vi "WM JONSWAP.vi"(3 "Sigma B":dbl=0.09 format="%.2f", 4 "End Freq (Model Scale)":dbl=100.0 min=0.0 format="%.2f", 5 "Start Freq (Model Scale)":dbl min=0.0 format="%.2f", 6 "Gamma":dbl=3.3 min=-1.0 max=9.0 format="%.2f", 7 "Sigma A":dbl=0.07 format="%.2f", 8 "Number of Frequencies":i32=100 min=2, 9 "Scale Ratio":dbl=1.0 min=0.0 step=0.01 format="%.2f", 10 "Peak Wave Period":dbl=1.0 min=0.0 step=0.01 format="%.2f", 11 "Significant Wave Height":dbl=1.0 min=0.0 step=0.01 format="%.2f") -> (0 "Frequency":dbl[](array[numeric]) caption="Hz" format="%.2f", 1 "Spectral Energy":dbl[](array[numeric]) format="%.2f", 2 "JONSWAP parameters":T1 {"Scale Ratio" format="%.2f"; "Sigma B" format="%.2f"; "Sigma A" format="%.2f"; "Gamma" format="%.2f"; "Sig Wave Period" format="%.2f"; "Sig Wave Height" format="%.2f"})   [LabVIEW 2012]
panel:
  in  "Boolean":bool
  # "JONSWAP Wave Spectra"
  # "m  (Full Scale)"
  # "s  (Full Scale)"
  # ":1"
  # "Full Scale : Model Scale"
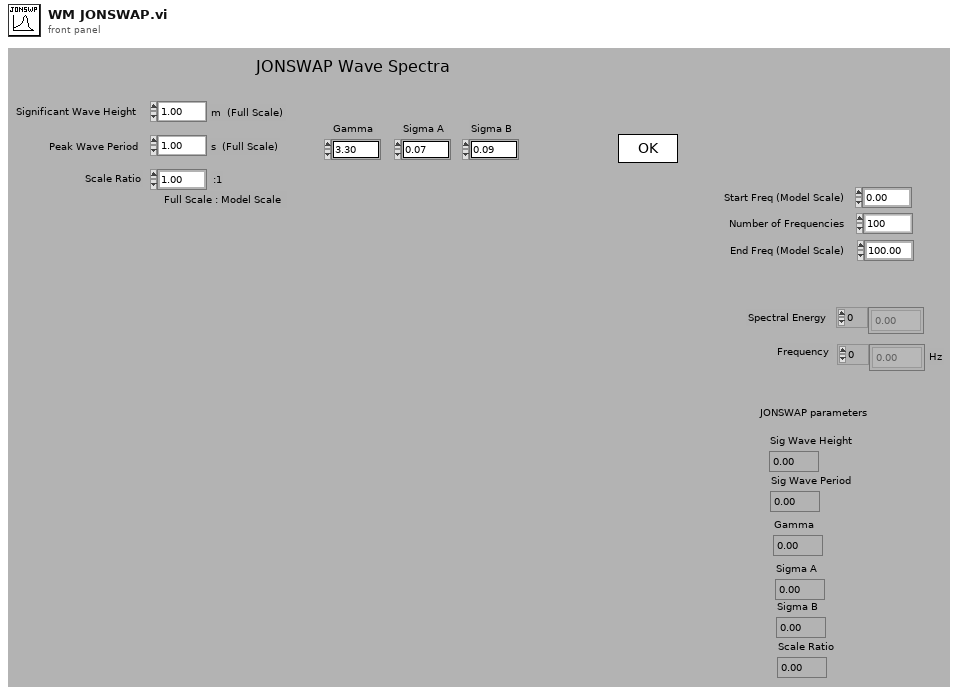
[diagram p1: front panel]
types:
  T1 = cluster{"Sig Wave Height":dbl, "Sig Wave Period":dbl, "Gamma":dbl, "Sigma A":dbl, "Sigma B":dbl, "Scale Ratio":dbl}
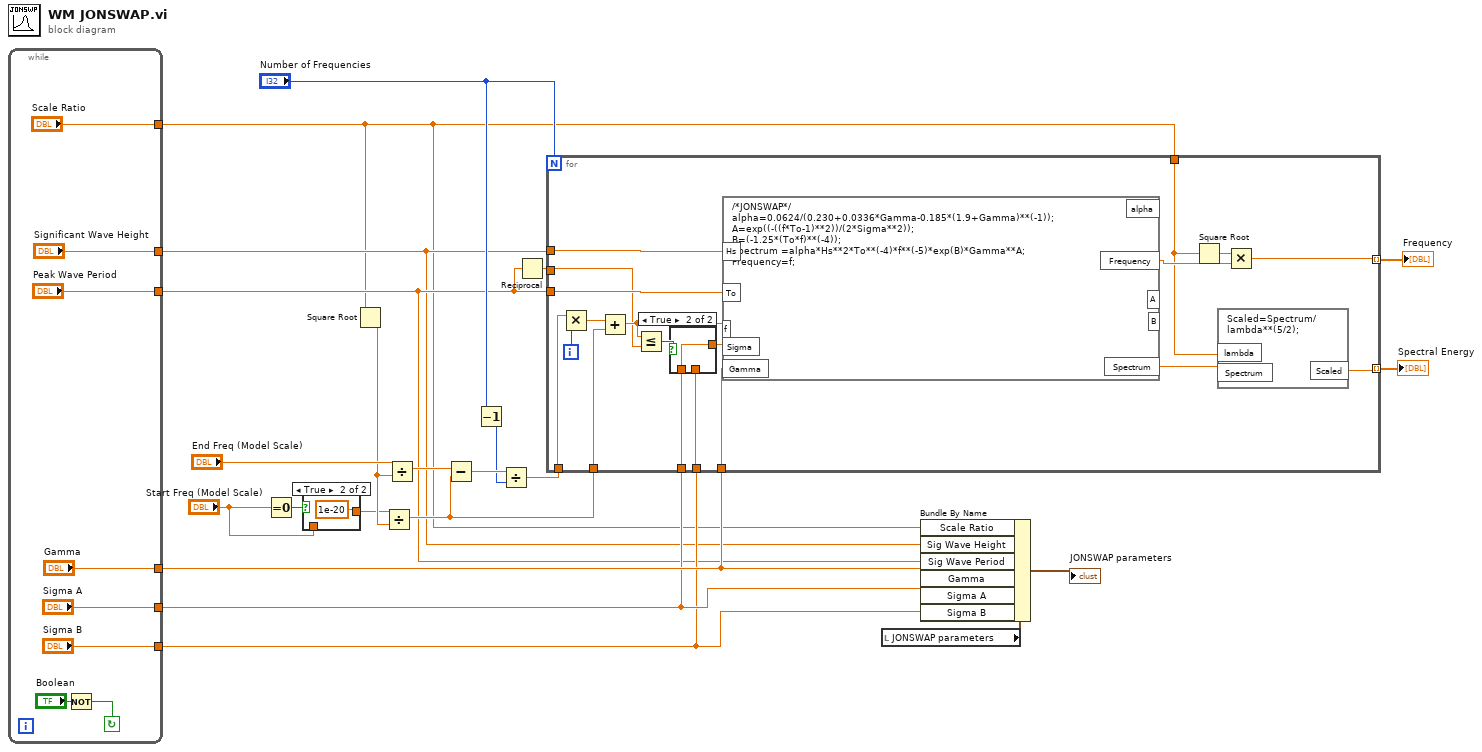
[diagram p0: block diagram]
diagram:
  n1 = while {
    tunnel: ["Scale Ratio"] -> w1
    tunnel: ["Significant Wave Height"] -> w2
    tunnel: ["Peak Wave Period"] -> w3
    tunnel: ["Sigma B"] -> w4
    tunnel: ["Sigma A"] -> w5
    tunnel: ["Gamma"] -> w6
    stop <- w23 continue-if-true
    n2 = Not(x="Boolean") -> (.not. x?=w23:bool)
  }
  n3 = Equal To 0?(x="Start Freq (Model Scale)") -> (x = 0?=w11:bool)
  n4 = case shown="True" w11 {
    tunnel: [w31 1e-20] -> w9
    tunnel: "Start Freq (Model Scale)" -> [w31 _]
    frame False {
    }
    frame True {
    }
  }
  n5 = Square Root(x=w1) -> (sqrt(x)=w14:dbl)
  n6 = Divide(x=w9, y=w14) -> (x/y=w13:dbl)
  n7 = Divide(x="End Freq (Model Scale)", y=w14) -> (x/y=w12:dbl)
  n8 = Subtract(x=w12, y=w13) -> (x-y=w19:dbl)
  n9 = Decrement(x="Number of Frequencies") -> (x-1=w16:i32)
  n10 = Divide(x=w19, y=w16) -> (x/y=w18:dbl)
  n11 = Reciprocal(x=w3) -> (1/x=w17:dbl)
  n12 = for {
    N: "Number of Frequencies" -> [_]
    tunnel: w2 -> [w40]
    tunnel: w3 -> [w42]
    tunnel: [w35] -> w22 mode=indexing
    tunnel: [w36] -> w21 mode=indexing
    tunnel: w13 -> [w38]
    tunnel: w18 -> [w49]
    tunnel: w17 -> [w41]
    tunnel: w5 -> [w47]
    tunnel: w4 -> [w46]
    tunnel: w6 -> [w45]
    tunnel: w1 -> [w34]
    i -> [w51]
    n13 = Multiply(x=w49, y=w51) -> (x*y=w39:dbl)
    n14 = Add(x=w39, y=w38) -> (x+y=w43:dbl)
    n15 = Less Or Equal?(x=w43, y=w41) -> (x <= y?=w48:bool)
    n16 = case shown="True" w48 {
      tunnel: w47 -> [_ w53]
      tunnel: w46 -> [w52 _]
      tunnel: [w52 w53] -> w44
      frame False {
      }
      frame True {
      }
    }
    n17 = formula code="/*JONSWAP*/\nalpha=0.0624/(0.230+0.0336*Gamma-0.185*(1.9+Gamma)**(-1));\nA=exp((-((f*To-1)**2))/(2*Sigma**2));\nB=(-1.25*(To*f)**(-4));\nSpectrum =alpha*Hs**2*To**(-4)*f**(-5)*exp(B)*Gamma**A;\nFrequency=f;"("Hs"=w40, "To"=w42, "f"=w43, "Sigma"=w44, "Gamma"=w45) -> ("Spectrum"=w37:dbl, "Frequency"=w50:dbl)  [unwired: 3 out]
    n18 = Square Root(x=w34) -> (sqrt(x)=w33:dbl)
    n19 = formula code="Scaled=Spectrum/lambda**(5/2);"("lambda"=w34, "Spectrum"=w37) -> ("Scaled"=w36:dbl)
    n20 = Multiply(x=w33, y=w50) -> (x*y=w35:dbl)
  }
  "Spectral Energy" <- w21
  "Frequency" <- w22
  n21 = local read "JONSWAP parameters"() -> (w8:T1)
  n22 = Bundle By Name(cluster=w8, "Scale Ratio"=w1, "Sig Wave Height"=w2, "Sig Wave Period"=w3, "Gamma"=w6, "Sigma A"=w5, "Sigma B"=w4) -> (→"JONSWAP parameters":T1)
